vi "RSZVB Set Number Of Stages.vi"(8 "error in (no error)":errorcluster {"code" format="%.0x"}, 9 "Number Of Stages (1)":i32=1, 10 "Channel (1)":i32=1, 11 "VISA resource name":refnum<visa-resource-name>) -> (0 "error out":errorcluster {"code" format="%.0x"}, 3 "VISA resource name out":refnum<visa-resource-name>)   [LabVIEW 2011]
doc: "Selects the number of converter/mixer stages for scalar mixer measurements and intermodulation distortion measurements.\n\nNotes:\n\nFor mixer delay measurements and vector mixer measurements (options R&S ZVA-K5, R&S ZVAK9, R&S ZVA-K10), a single mixer stage is supported only.\n\nRemote-control command(s):\n[SENSe<Ch>:]FREQuency:CONVersion:MIXer:STAGes <mixers>"
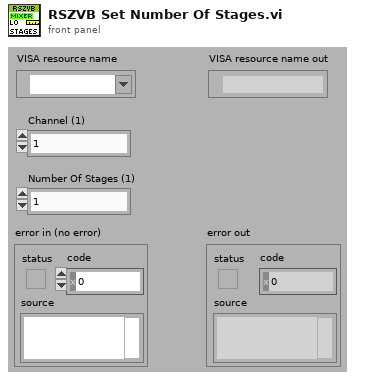
[diagram p1: front panel]
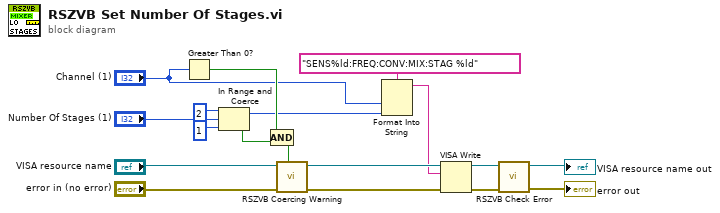
[diagram p0: block diagram]
diagram:
  n1 = Greater Than 0?(x="Channel (1)") -> (x > 0?=w11:bool)
  n2 = In Range and Coerce(upper limit=2, x="Number Of Stages (1)", lower limit=1) -> (coerced(x)=w1:i32, In Range?=w12:bool)
  n3 = Compound Arithmetic op=AND(w11, w12) -> (w10:bool)
  n4 = call "RSZVB Coercing Warning.vi"("In Range?"=w10, "error in (no error)"="error in (no error)", "VISA session"="VISA resource name") -> ("error out"=w15:errorcluster, "dup VISA session"=w16:refnum<visa-resource-name>)  [unwired: 7 in]
  n5 = Format Into String(format string="SENS%ld:FREQ:CONV:MIX:STAG %ld", "Channel (1)", w1) -> (resulting string=w3:string)  [unwired: 2 in, 1 out]
  n6 = VISA Write(VISA resource name=w16, write buffer=w3, error in (no error)=w15) -> (VISA resource name out=w13:refnum<visa-resource-name>, error out=w14:errorcluster)  [unwired: 1 out]
  n7 = call "RSZVB Check Error.vi"("error in (no error)"=w14, "VISA session"=w13) -> ("error out"=→"error out":errorcluster, "dup VISA session"=→"VISA resource name out":refnum<visa-resource-name>)  [unwired: 8 in]
